vi "MakePlantUML.vi"(4 "ShowLegend":bool=TRUE, 6 "Orientation":enum16{"Horizonal", "Vertical"}(ring), 7 "DiagramName":string, 9 "Simplified":bool, 10 "NavigationsDetails":cluster{T2[]}[](array[cluster]), 11 "NavigationNames":string[](array[string])) -> (2 "Uniques":T1, 3 "PlantUMLText":string)   [LabVIEW 2021, in "ButtonBarFlow.lvlib"]
uses:
  ButtonBarFlow.lvlib
  ActiveObjects/VerticalButtonBar/ButtonCollection/ButtonDefinition.ctl
  ActiveObjects/VerticalButtonBar/ButtonCollection/ButtonCollection.lvclass
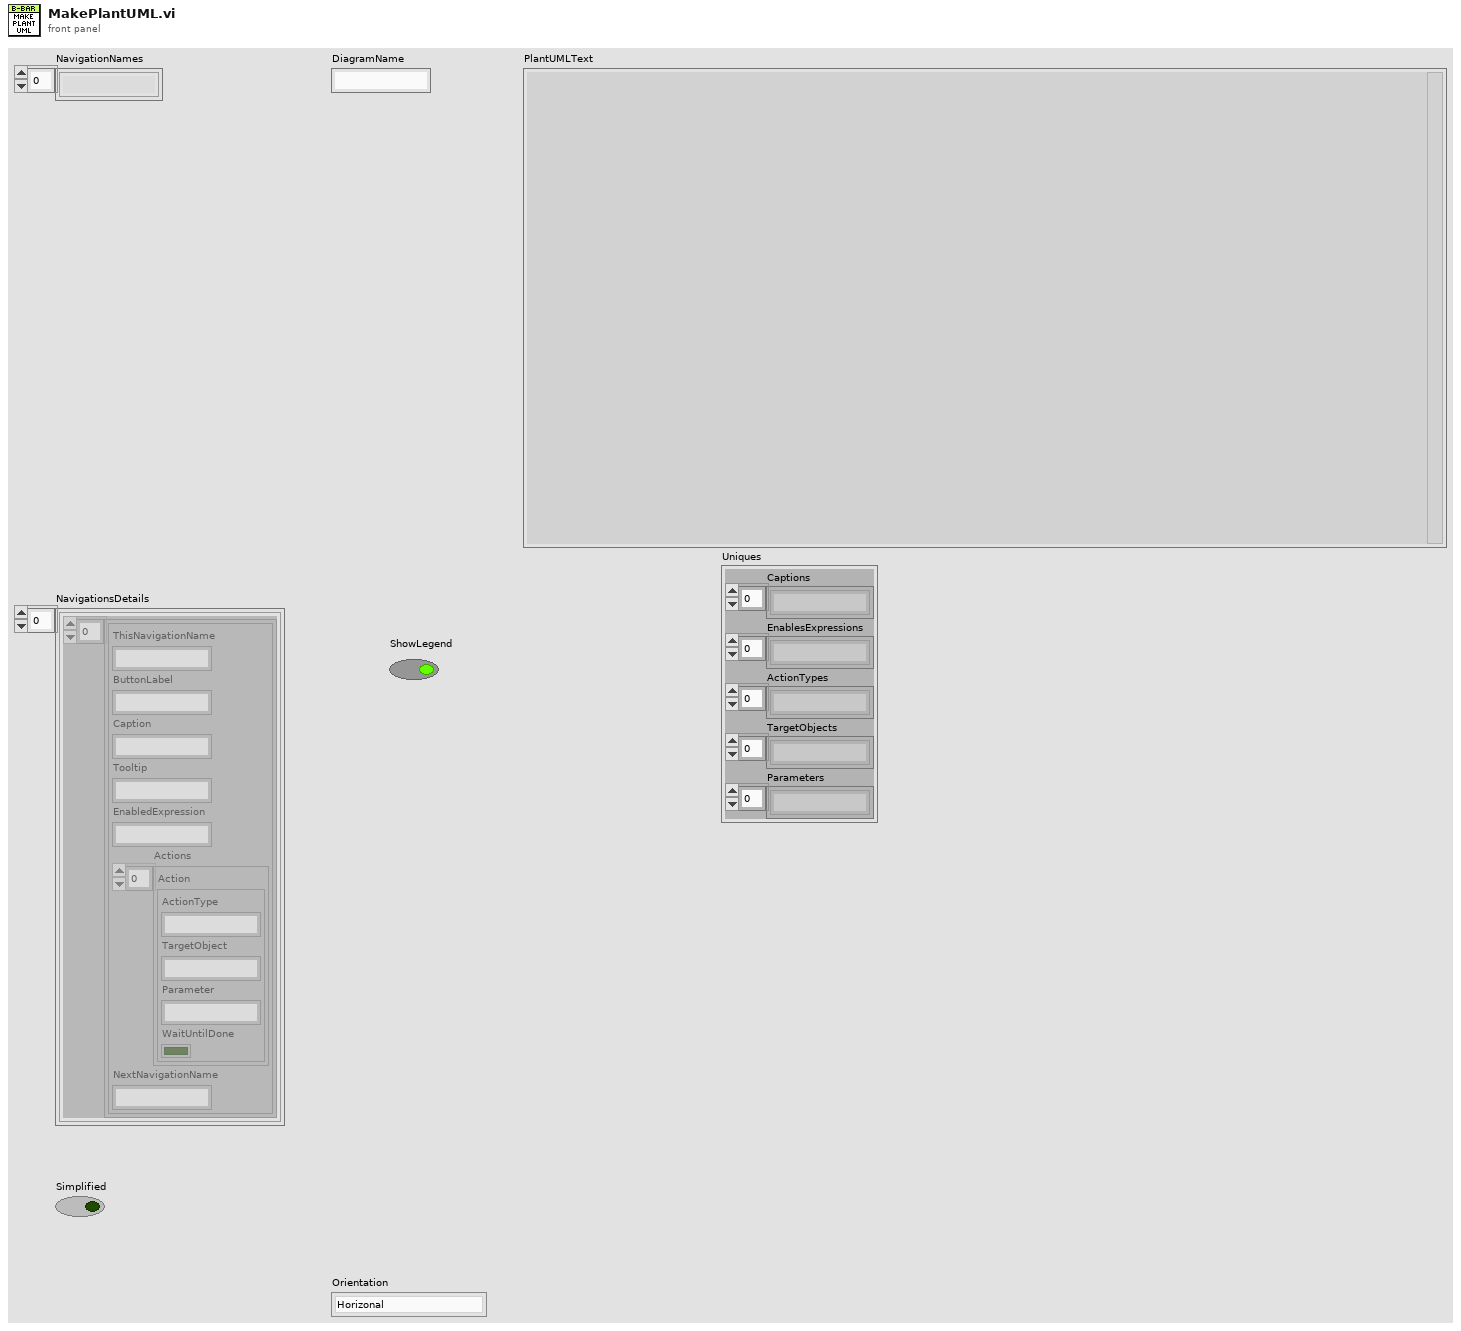
[diagram p1: front panel]
types:
  T1 = cluster{"Captions":string[], "EnablesExpressions":string[], "ActionTypes":string[], "TargetObjects":string[], "Parameters":string[]}
  T2 = typedef "ButtonCollection.lvclass/ButtonDefinition.ctl" = cluster{"ThisNavigationName":string, "ButtonLabel":string, "Caption":string, "Tooltip":string, "EnabledExpression":string, "Actions":cluster{"ActionType":string, "TargetObject":string, "Parameter":string, "WaitUntilDone":bool}[], "NextNavigationName":string}
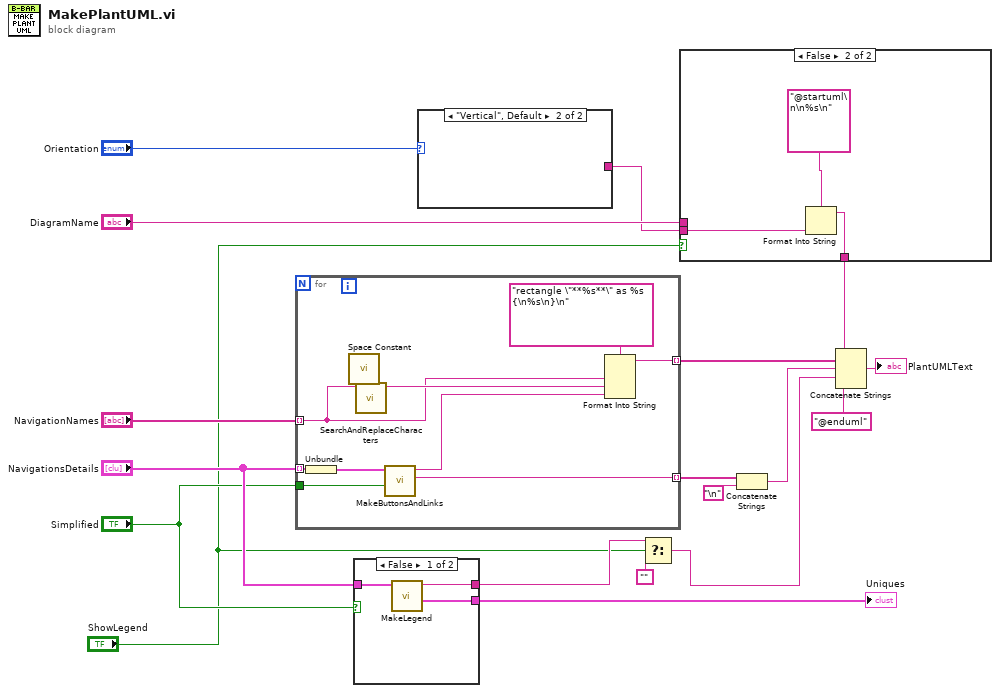
[diagram p0: block diagram]
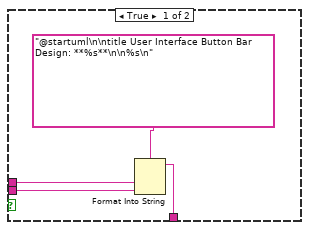
[diagram p2: hidden frame]
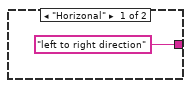
[diagram p4: hidden frame]
diagram:
  n1 = for {
    tunnel: "NavigationNames" -> [w22] mode=indexing
    tunnel: "NavigationsDetails" -> [w27] mode=indexing
    tunnel: [w26] -> w14 mode=indexing
    tunnel: [w20] -> w11 mode=indexing
    tunnel: "Simplified" -> [w19]
    n2 = Unbundle(w27) -> (w24:T2[])
    n3 = call <vilib>:"Space Constant.vi"() -> ("String"=w23:string)
    n4 = call "SearchAndReplaceCharacters.vi"("CharactersToSearch"=w23, "StringIn"=w22) -> ("ResultString"=w25:string)  [unwired: 9 in]
    n5 = call "MakeButtonsAndLinks.vi"("Simplified"=w19, "Nagivations"=w24) -> ("Links"=w20:string, "Buttons"=w21:string)  [unwired: 8 in]
    n6 = Format Into String(format string="rectangle \"**%s**\" as %s {\n%s\n}\n", w22, w25, w21) -> (resulting string=w26:string)  [unwired: 2 in, 1 out]
  }
  n7 = case shown="False" "Simplified" {
    tunnel: "NavigationsDetails" -> [w31 _]
    tunnel: [w30 _] -> w4
    tunnel: [w29 _] -> w5
    frame False {
      n8 = call "MakeLegend.vi"("NavigationsDetails"=w31) -> ("Uniques"=w29:T1, "PlantUMLText"=w30:string)  [unwired: 9 in]
    }
    frame True {
    }
  }
  "Uniques" <- w5
  n9 = case shown="\"Vertical\", Default" "Orientation" {
    tunnel: ["left to right direction" _] -> w6
    frame "Horizonal" {
    }
    frame "Vertical", Default {
    }
  }
  n10 = Select(t=w4, s="ShowLegend", f="") -> (s? t:f=w3:string)
  n11 = case shown="False" "ShowLegend" {
    tunnel: [w36 w39] -> w17
    tunnel: "DiagramName" -> [w35 _]
    tunnel: w6 -> [w33 w37]
    frame True {
      n12 = Format Into String(format string="@startuml\n\ntitle User Interface Button Bar Design: **%s**\n\n%s\n", w35, w33) -> (resulting string=w36:string)  [unwired: 2 in, 1 out]
    }
    frame False {
      n13 = Format Into String(format string="@startuml\n\n%s\n", w37) -> (resulting string=w39:string)  [unwired: 2 in, 1 out]
    }
  }
  n14 = Concatenate Strings(w11, "\n") -> (w10:string)
  n15 = Concatenate Strings(w17, w14, w10, w3, "@enduml" ("format string")) -> (→"PlantUMLText":string)
